vi "Agilent N6700 Series Configure Histogram.vi"() -> ()   [LabVIEW 2016]
doc: "Configure the histogram, histogram trigger source, initiates the histogram, triggers the histogram and fetches the histogram bin data.\n\n<b>Note:</b>\n\nThis VI only applies to the N6705B and N6705C DC Power Analyzer."
uses:
  <instrlib>/Agilent N6700 Series/Agilent N6700 Series.lvlib
panel:
  in  "Enable Histogram (True)":bool
  in  "Wait Time (1000 ms)":i32=1000
  out "Bin Data":dbl[](array[numeric]) format="%^.3e"
  in  "Histogram Trigger Source (1: Software)":i32(ring)=1 items=["External", "Software", "Immediate", "Pin 1", "Pin 2", "Pin 3"]
  in  "Histogram Range (0.0)":dbl format="%^.3e"
  in  "Bin Range (0: 8 A)":i32(ring) items=["8 A", "0.0039 A"]
  in  "Channel Name (1)":string="1"
  in  "VISA resource name":refnum<visa-resource-name>
  # "(c) 2012-2019  National Instruments.  ALL RIGHTS RESERVED."
  # "Agilent N6705 DC Power Supply"
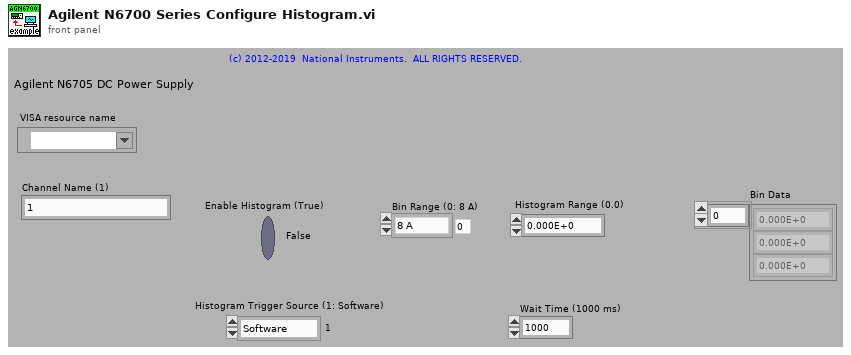
[diagram p1: front panel]
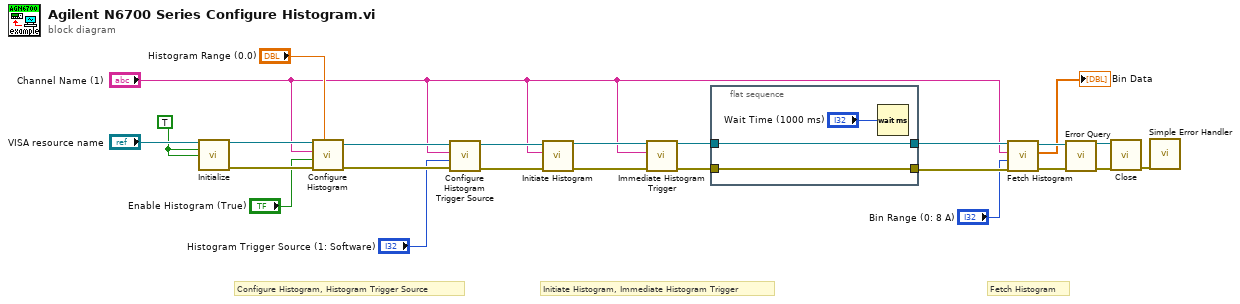
[diagram p0: block diagram]
diagram:
  w22 = TRUE ("Reset? (T: Yes)")
  # "Fetch Histogram"
  # "Initiate Histogram, Immediate Histogram Trigger"
  # "Configure Histogram, Histogram Trigger Source"
  n1 = call <instrlib>:"Initialize.vi"("VISA resource name"="VISA resource name", "ID Query? (T: Yes)"=w22, "Reset? (T: Yes)"=w22) -> ("VISA resource name out"=w18:refnum<visa-resource-name>, "error out"=w17:errorcluster)  [unwired: 11 in]
  n2 = call <instrlib>:"Configure Histogram.vi"("Histogram Range (0.0)"="Histogram Range (0.0)", "error in (no error)"=w17, "Enable Histogram (False)"="Enable Histogram (True)", "Channel Name (1)"="Channel Name (1)", "VISA resource name"=w18) -> ("error out"=w16:errorcluster, "VISA resource name out"=w15:refnum<visa-resource-name>)  [unwired: 5 in]
  n3 = call <instrlib>:"Configure Histogram Trigger Source.vi"("error in (no error)"=w16, "Histogram Trigger Source (1: Software)"="Histogram Trigger Source (1: Software)", "Channel Name (1)"="Channel Name (1)", "VISA resource name"=w15) -> ("error out"=w7:errorcluster, "VISA resource name out"=w8:refnum<visa-resource-name>)  [unwired: 6 in]
  n4 = call <instrlib>:"Initiate Histogram.vi"("error in (no error)"=w7, "Channel Name (1)"="Channel Name (1)", "VISA resource name"=w8) -> ("error out"=w6:errorcluster, "VISA resource name out"=w9:refnum<visa-resource-name>)  [unwired: 7 in]
  n5 = call <instrlib>:"Immediate Histogram Trigger.vi"("error in (no error)"=w6, "Channel Name (1)"="Channel Name (1)", "VISA resource name"=w9) -> ("error out"=w4:errorcluster, "VISA resource name out"=w5:refnum<visa-resource-name>)  [unwired: 7 in]
  n6 = flat-sequence {
    tunnel: w4 -> [w28]
    tunnel: [w28] -> w13
    tunnel: w5 -> [w27]
    tunnel: [w27] -> w14
    frame #0 {
      n7 = Wait (ms)(milliseconds to wait="Wait Time (1000 ms)") -> ()  [unwired: 1 out]
    }
  }
  n8 = call <instrlib>:"Fetch Histogram.vi"("error in (no error)"=w13, "Bin Range (0: 8A)"="Bin Range (0: 8 A)", "Channel Name (1)"="Channel Name (1)", "VISA resource name"=w14) -> ("error out"=w24:errorcluster, "Bin Data"=→"Bin Data":dbl[], "VISA resource name out"=w25:refnum<visa-resource-name>)  [unwired: 5 in]
  n9 = call <instrlib>:"Error Query.vi"("VISA resource name"=w25, "error in (no error)"=w24) -> ("VISA resource name out"=w19:refnum<visa-resource-name>, "error out"=w20:errorcluster)  [unwired: 10 in, 2 out]
  n10 = call <instrlib>:"Close.vi"("VISA resource name"=w19, "error in (no error)"=w20) -> ("error out"=w21:errorcluster)  [unwired: 13 in]
  n11 = call <vilib>:"Simple Error Handler.vi"("error in (no error)"=w21) -> ()  [unwired: 4 in, 5 out]
